vi "Initialize.vi"(8 "error in":errorcluster) -> (0 "error out":errorcluster)   [LabVIEW 2020, in "GUI.lvlib"]
uses:
  GUI.lvlib
  Eventing/Event FGV Actions.ctl
panel:
  # "Event Handler: Initialize"
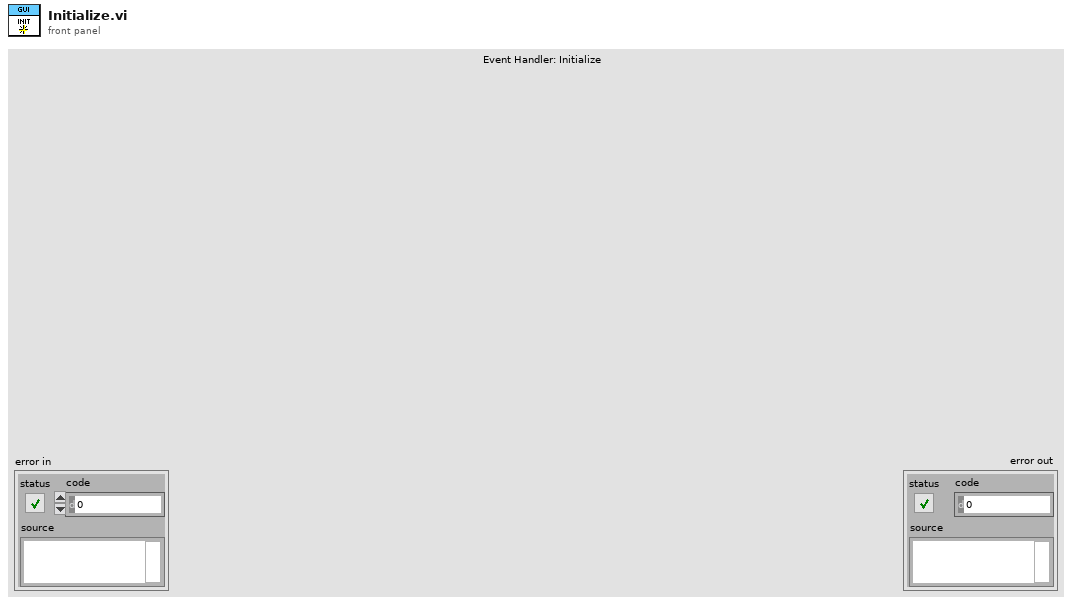
[diagram p1: front panel]
types:
  T1 = typedef "GUI.lvlib/Event FGV Actions.ctl" = enum16{"Get", "Create", "Destroy"}
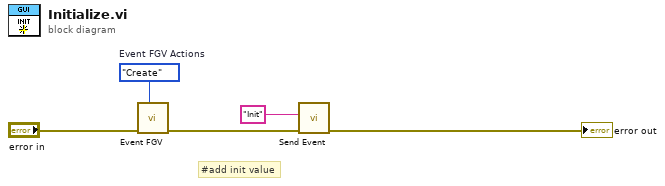
[diagram p0: block diagram]
diagram:
  w5 = Event_FGV_Actions."Create"  # Event FGV Actions
  # "#add init value"
  n1 = call "Event FGV.vi"("Event FGV Actions"=w5, "error in"="error in") -> ("error out"=w2:errorcluster)  [unwired: 7 in, 2 out]
  n2 = call "Send Event.vi"("error in"=w2, "Command"="Init") -> ("error out"=→"error out":errorcluster)  [unwired: 9 in]
